vi "Schedule Obsidian Robot.vi"(6 "max geodes in":u8=24, 7 "max time in":u8=24, 8 "costs in":T1, 9 "data value reference":refnum<data-value>, 10 "stack in":refnum<queue>, 11 "mine in":refnum<class "Mine.lvclass">) -> (0 "costs out":T1, 1 "data value reference":refnum<data-value>, 2 "stack out":refnum<queue>, 3 "mine out":refnum<class "Mine.lvclass">, 4 "max geodes out":u8, 5 "max time out":u8)   [LabVIEW 2023, in "d19.lvlib" / "Mine.lvclass"]
uses:
  Mine.lvclass
  Mine.lvclass/Mine.ctl
  <vilib>/Utility/miscctls.llb/LVMapReplaceAction.ctl
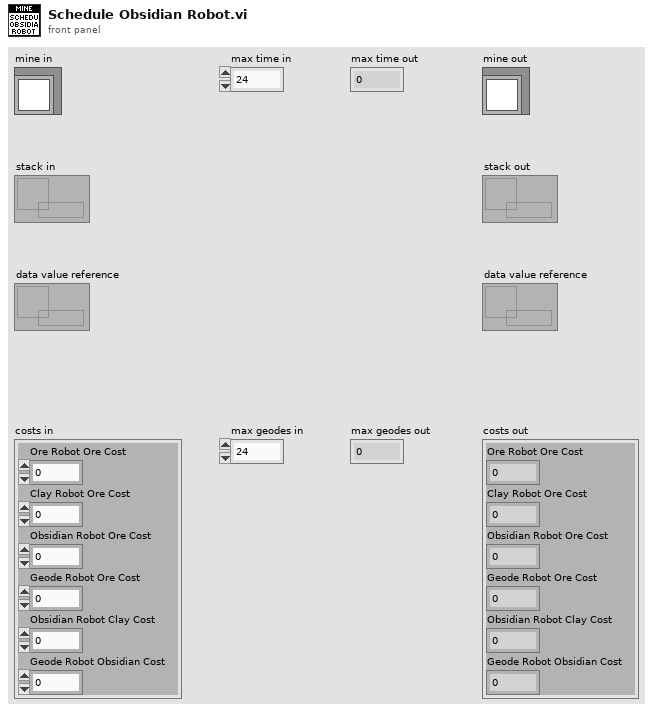
[diagram p1: front panel]
types:
  T1 = cluster{"Ore Robot Ore Cost":u8, "Clay Robot Ore Cost":u8, "Obsidian Robot Ore Cost":u8, "Geode Robot Ore Cost":u8, "Obsidian Robot Clay Cost":u8, "Geode Robot Obsidian Cost":u8}
  T2 = typedef "LVMapReplaceAction.ctl" = enum32{"Modify Entry only if found", "Add or Modify Entry", "Delete Entry"}
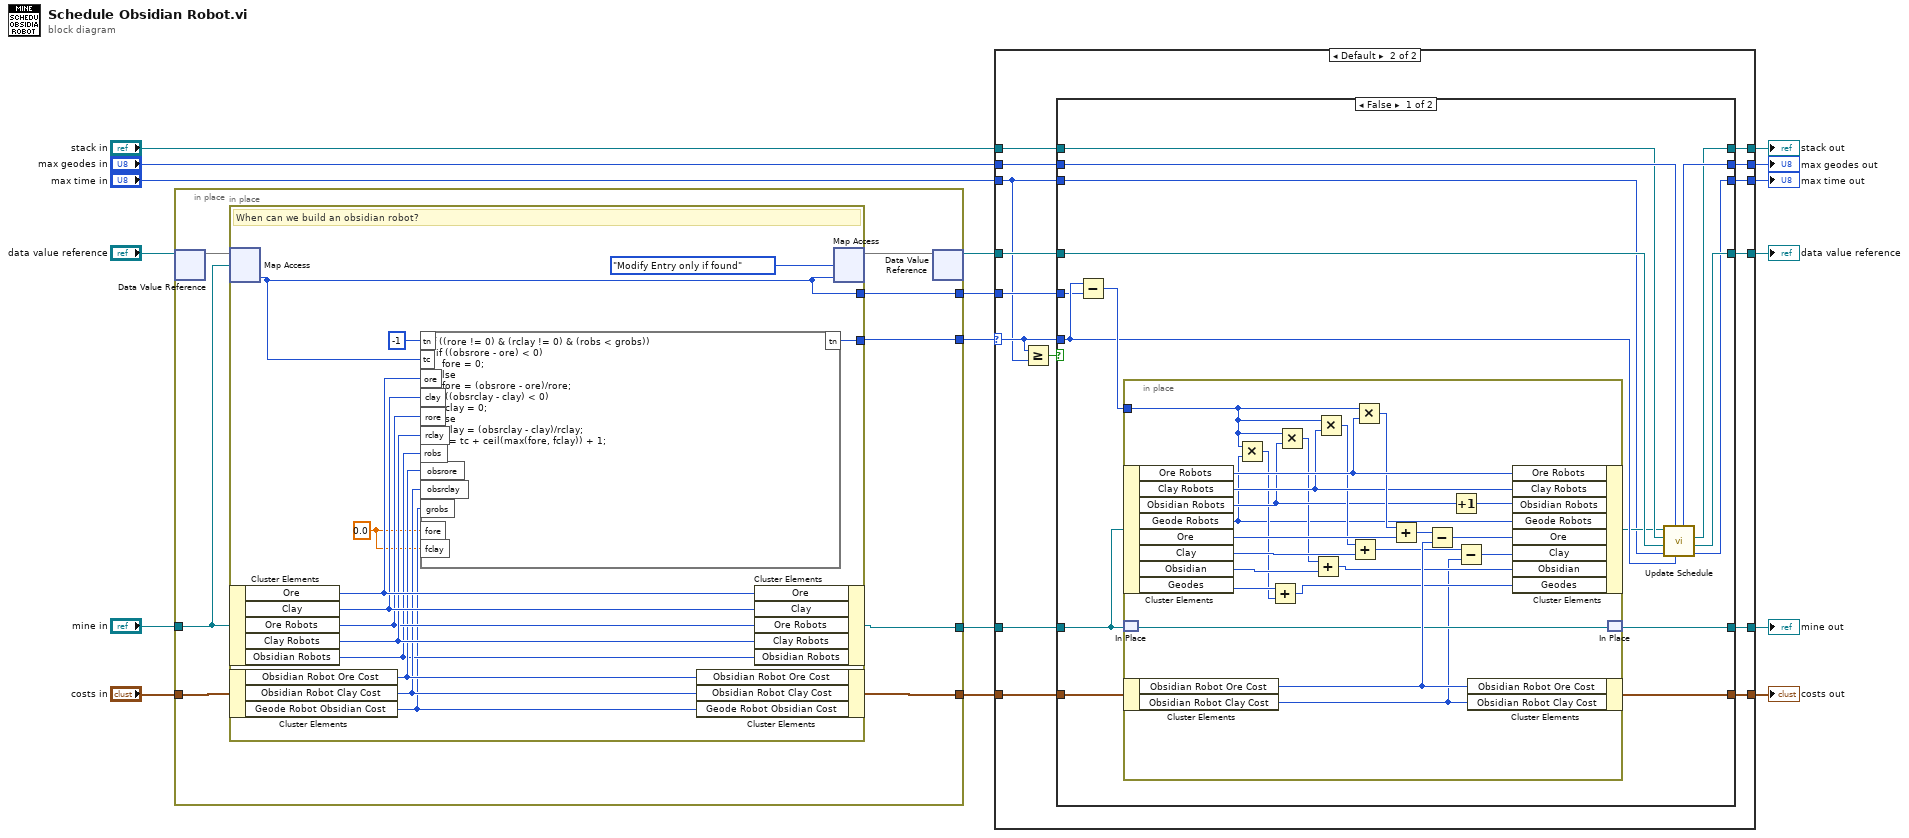
[diagram p0: block diagram]
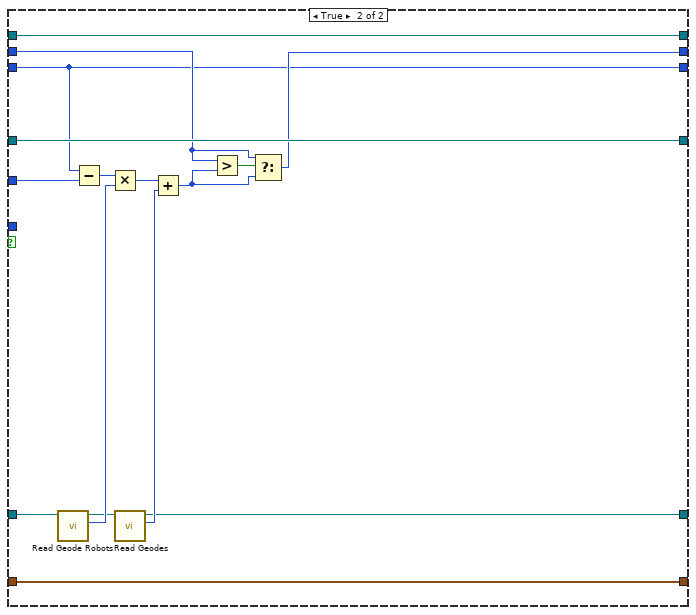
[diagram p3: hidden frame]
diagram:
  n1 = in-place {
    in-place-border: "costs in" -> [w25]
    in-place-border: "mine in" -> [w24]
    in-place-border: [w23] -> w15
    in-place-border: [w22] -> w11
    in-place-border: [w21] -> w10
    in-place-border: [w20] -> w6
    n2 = in-place-dvr #1("data value reference") -> (w19:map{refnum<class "Mine.lvclass">, u8})  [unwired: 1 out]
    n3 = in-place {
      in-place-border: [w30] -> w23
      in-place-border: [w26] -> w20
      w27 = 0.0 ("input variable")
      # "When can we build an obsidian robot?"
      n4 = in-place-map #2(w19, w24) -> (w26:u8)  [unwired: 1 in, 1 out]
      n5 = in-place-cluster #3(w24) -> ("Ore"=w37:u8, "Clay"=w36:u8, "Ore Robots"=w34:u8, "Clay Robots"=w35:u8, "Obsidian Robots"=w29:u8)
      n6 = in-place-cluster #4(w25) -> ("Obsidian Robot Ore Cost"=w33:u8, "Obsidian Robot Clay Cost"=w32:u8, "Geode Robot Obsidian Cost"=w28:u8)
      n7 = formula code="if ((rore != 0) & (rclay != 0) & (robs < grobs))\n  if ((obsrore - ore) < 0)\n    fore = 0;\n  else\n    fore = (obsrore - ore)/rore;\n  if ((obsrclay - clay) < 0)\n    fclay = 0;\n  else\n    fclay = (obsrclay - clay)/rclay;\n  tn = tc + ceil(max(fore, fclay)) + 1;"("tc"=w26, "obsrore"=w33, "obsrclay"=w32, "ore"=w37, "clay"=w36, "rore"=w34, "rclay"=w35, "tn"=i8 -1, "robs"=w29, "grobs"=w28, "fore"=w27, "fclay"=w27) -> ("tn"=w30:i8)
      n8 = in-place-cluster #4("Obsidian Robot Ore Cost"=w33, "Obsidian Robot Clay Cost"=w32, "Geode Robot Obsidian Cost"=w28) -> (w22:T1)
      n9 = in-place-cluster #3("Ore"=w37, "Clay"=w36, "Ore Robots"=w34, "Clay Robots"=w35, "Obsidian Robots"=w29) -> (w21:refnum<class "Mine.lvclass">)
      n10 = in-place-map #2(w26, LVMapReplaceAction."Modify Entry only if found" ("action")) -> (w18:map{refnum<class "Mine.lvclass">, u8})  [unwired: 2 out]
    }
    n11 = in-place-dvr #1(w18) -> (w1:refnum<data-value>)  [unwired: 1 out]
  }
  n12 = case shown="Default" w15 {
    selector: w15 -> [_ w47]
    tunnel: "stack in" -> [w44 w59]
    tunnel: [w44 w58] -> w13
    tunnel: [w41 w57] -> w12
    tunnel: w11 -> [w39 w56]
    tunnel: w10 -> [w40 w55]
    tunnel: [w39 w54] -> w9
    tunnel: [w40 w53] -> w8
    tunnel: "max time in" -> [w42 w46]
    tunnel: w6 -> [_ w52]
    tunnel: "max geodes in" -> [w43 w51]
    tunnel: [w43 w50] -> w4
    tunnel: [w42 w49] -> w3
    tunnel: w1 -> [w41 w48]
    frame -1 {
    }
    frame Default {
      n13 = Greater Or Equal?(x=w47, y=w46) -> (x >= y?=w45:bool)
      n14 = case shown="False" w45 {
        tunnel: w48 -> [w65 w114]
        tunnel: [w62 w114] -> w57
        tunnel: w59 -> [w66 w113]
        tunnel: [w61 w113] -> w58
        tunnel: w56 -> [w75 w112]
        tunnel: w55 -> [w72 w101]
        tunnel: [w74 w112] -> w54
        tunnel: [w71 w99] -> w53
        tunnel: w46 -> [w63 w107]
        tunnel: w52 -> [w67 w106]
        tunnel: w51 -> [w70 w109]
        tunnel: [w69 w110] -> w50
        tunnel: [w60 w107] -> w49
        tunnel: w47 -> [w68 _]
        frame False {
          n15 = Subtract(x=w68, y=w67) -> (x-y=w73:u8)
          n16 = in-place {
            in-place-border: w73 -> [w82]
            n17 = in-place-cluster #5(w72) -> ("Ore Robots"=w92:u8, "Clay Robots"=w88:u8, "Obsidian Robots"=w86:u8, "Geode Robots"=w80:u8, "Ore"=w98:u8, "Clay"=w95:u8, "Obsidian"=w85:u8, "Geodes"=w94:u8)
            n18 = in-place-match #6(w72) -> (w93:refnum<class "Mine.lvclass">)
            n19 = in-place-cluster #7(w75) -> ("Obsidian Robot Ore Cost"=w97:u8, "Obsidian Robot Clay Cost"=w76:u8)
            n20 = Multiply(x=w82, y=w80) -> (x*y=w81:u8)
            n21 = Add(x=w94, y=w81) -> (x+y=w79:u8)
            n22 = Multiply(x=w82, y=w86) -> (x*y=w83:u8)
            n23 = Add(x=w83, y=w85) -> (x+y=w84:u8)
            n24 = Multiply(x=w82, y=w88) -> (x*y=w87:u8)
            n25 = Add(x=w87, y=w95) -> (x+y=w90:u8)
            n26 = Multiply(x=w82, y=w92) -> (x*y=w89:u8)
            n27 = Add(x=w89, y=w98) -> (x+y=w91:u8)
            n28 = Subtract(x=w91, y=w97) -> (x-y=w96:u8)
            n29 = Increment(x=w86) -> (x+1=w78:u8)
            n30 = Subtract(x=w90, y=w76) -> (x-y=w77:u8)
            n31 = in-place-cluster #7("Obsidian Robot Ore Cost"=w97, "Obsidian Robot Clay Cost"=w76) -> (w74:T1)
            n32 = in-place-cluster #5("Ore Robots"=w92, "Clay Robots"=w88, "Obsidian Robots"=w78, "Geode Robots"=w80, "Ore"=w96, "Clay"=w77, "Obsidian"=w84, "Geodes"=w79) -> (w64:refnum<class "Mine.lvclass">)
            n33 = in-place-match #6(w93) -> (w71:refnum<class "Mine.lvclass">)
          }
          n34 = call "Update Schedule.vi"("new time"=w68, "max geodes in"=w70, "max time in"=w63, "map in"=w65, "stack in"=w66, "Mine in"=w64) -> ("max time out"=w60:u8, "map out"=w62:refnum<data-value>, "stack out"=w61:refnum<queue>, "max geodes out"=w69:u8)  [unwired: 1 in, 1 out]
        }
        frame True {
          n35 = call "Read Geode Robots.vi"("Mine in"=w101) -> ("Geode Robots"=w104:u8, "Mine out"=w100:refnum<class "Mine.lvclass">)  [unwired: 9 in]
          n36 = Subtract(x=w107, y=w106) -> (x-y=w105:u8)
          n37 = Multiply(x=w105, y=w104) -> (x*y=w103:u8)
          n38 = call "Read Geodes.vi"("Mine in"=w100) -> ("Geodes"=w108:u8, "Mine out"=w99:refnum<class "Mine.lvclass">)  [unwired: 9 in]
          n39 = Add(x=w103, y=w108) -> (x+y=w102:u8)
          n40 = Greater?(x=w109, y=w102) -> (0:w111:bool)
          n41 = Select(t=w109, s=w111, f=w102) -> (s? t:f=w110:u8)
        }
      }
    }
  }
  "stack out" <- w13
  "data value reference" <- w12
  "costs out" <- w9
  "mine out" <- w8
  "max geodes out" <- w4
  "max time out" <- w3
